vi "Read Writer.vi"(8 "Error In":errorcluster, 11 "Renderer In":refnum<class "Renderer.lvclass">) -> (0 "Error Out":errorcluster, 2 "Writer":refnum<class "Writer.lvclass">, 3 "Renderer Out":refnum<class "Renderer.lvclass">)   [LabVIEW 2018, in "Toolkit.lvlib" / "Renderer.lvclass"]
uses:
  Renderer.lvclass
  Writers/Writer/Writer.lvclass
  Renderer.lvclass/Renderer.ctl
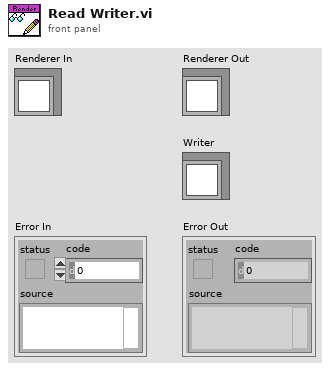
[diagram p1: front panel]
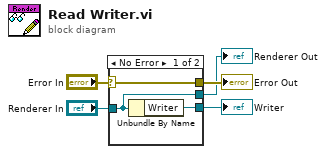
[diagram p0: block diagram]
diagram:
  n1 = case shown="No Error" "Error In" {
    selector: "Error In" -> [w8 w9]
    tunnel: [w8 w9] -> w4
    tunnel: [w7 w10] -> w2
    tunnel: "Renderer In" -> [w7 w10]
    tunnel: [w6 _] -> w1
    frame No Error {
      n2 = Unbundle By Name(w7) -> ("Writer"=w6:refnum<class "Writer.lvclass">)
    }
    frame Error {
    }
  }
  "Error Out" <- w4
  "Renderer Out" <- w2
  "Writer" <- w1
